vi "NR_RS_Gen.vi"(2 "prb_num":dbl, 3 "Second_DMRS_L":dbl, 4 "Frist_DMRS_L0":dbl, 5 "TransformPrcode_en":dbl, 6 "UL_DMRS_Config_type":dbl, 7 "beltaDMRS":dbl, 8 "error in (no error)":errorcluster caption="错误输入（无错误）", 9 "nslotnum":dbl, 10 "cellid":dbl, 11 "appended path":path) -> (0 "error IO":errorcluster, 1 "rsdata":cdb[][](array[numeric]))   [LabVIEW 2015]
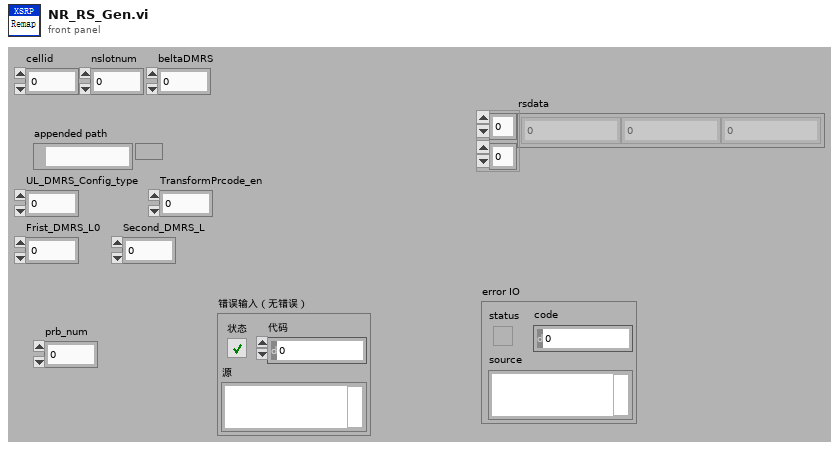
[diagram p1: front panel]
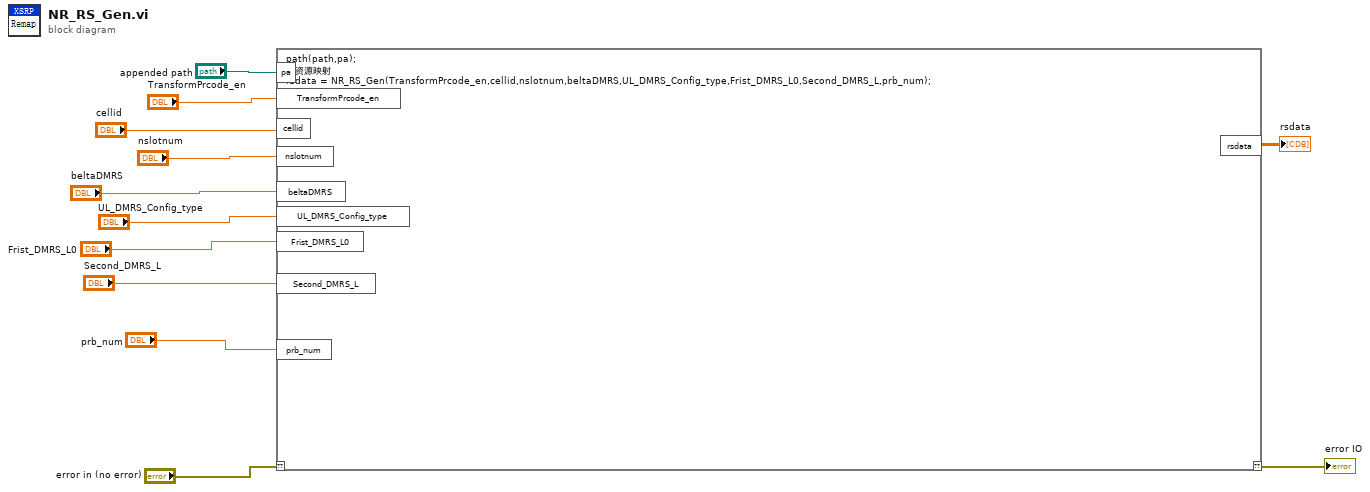
[diagram p0: block diagram]
diagram:
  n1 = script code="path(path,pa);\n%资源映射\nrsdata = NR_RS_Gen(TransformPrcode_en,cellid,nslotnum,beltaDMRS,UL_DMRS_Config_type,Frist_DMRS_L0,Second_DMRS_L,prb_num);"("??"="error in (no error)", "pa"="appended path", "cellid"="cellid", "nslotnum"="nslotnum", "beltaDMRS"="beltaDMRS", "prb_num"="prb_num", "TransformPrcode_en"="TransformPrcode_en", "UL_DMRS_Config_type"="UL_DMRS_Config_type", "Frist_DMRS_L0"="Frist_DMRS_L0", "Second_DMRS_L"="Second_DMRS_L") -> ("??"=→"error IO":errorcluster, "rsdata"=→"rsdata":cdb[][])
